vi "Create.vi"(9 "Encoding":T1, 10 "Statement handle":u64, 11 "SQLite dll":path) -> (3 "SQL Statement out":refnum<class "SQL Statement.lvclass">)   [LabVIEW 2011, in "SQLite.lvlib" / "SQL Statement.lvclass"]
uses:
  SQL Statement.lvclass
  SQL Statement.lvclass/SQL Statement.ctl
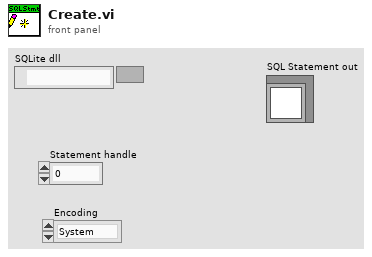
[diagram p1: front panel]
types:
  T1 = typedef "SQLite.lvlib/SQL Statement.lvclass/Text Encoding" = enum16{"System", "UTF-8", "UTF-16"}
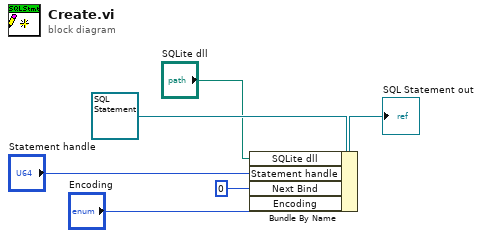
[diagram p0: block diagram]
diagram:
  n1 = Bundle By Name(cluster=refnum<class "SQL Statement.lvclass"> refnum ("SQL Statement in"), "SQLite dll"="SQLite dll", "Statement handle"="Statement handle", "Next Bind"=0, "Encoding"="Encoding") -> (→"SQL Statement out":refnum<class "SQL Statement.lvclass">)
